vi "Positioncontrol_twomotor_pid_MotorID.vi"() -> ()   [LabVIEW 2014]
uses:
  <vilib>/rvi/FXPMathLib/FxpSinAndCos/subVIs/nifxpmath_SinAndCos_SimConfig.ctl
  <vilib>/rvi/Emulation/niFpgaGetClockAttributes.vi
  <vilib>/rvi/Emulation/niFpgaSctlEmulationGetInTimedLoop.vi
  <vilib>/rvi/Emulation/niFpgaEmulationReportErrorSimple.vi
  <vilib>/rvi/Emulation/niFpgaProcessEmulError.vi
  <vilib>/rvi/FXPMathLib/FxpSinAndCos/simVIs/DllFxpSinAndCosTemp_sub.vi
  <vilib>/rvi/Emulation/niFpgaCriticalErrorInLSC.vi
  <vilib>/rvi/eio/common/nirviEmuTemplateMethod_errors.vi
  <vilib>/rvi/interface/RandomDataEmulation/nirviRandomDataMultiElementFPGAFIFO.vi
  <instcachedir>/0/nirviRandomDataMultiElementFPGAFIFO_AD0CFC12EF974623A9C2E4184BC062B2.lvgen/nirviRandomDataMultiElementFPGAFIFO_AD0CFC12EF974623A9C2E4184BC062B2_004.vi
  <vilib>/rvi/interface/RandomDataEmulation/niFpgaRandomDataHandleErrors.vi
  <vilib>/rvi/FXPMathLib/FxpSinAndCos/XNode/nifxpmath_SinAndCos.xnode
  <vilib>/eio/EIONode/EIONode.xnode
  <vilib>/rvi/FXPMathLib/FxpMul/XNode/nifxpmath_Multiplier.xnode
  <vilib>/rvi/FXPMathLib/FxpSub/XNode/nifxpmath_Sub.xnode
  <vilib>/rvi/FXPMathLib/FxpAdd/XNode/nifxpmath_Add.xnode
  <vilib>/rvi/Analysis/measure/butterworth/XNode/niFpgaButterworthFilter.xnode
  <vilib>/rvi/DataTransferAndStorage/Container/XNode/niFpgaContainer.xnode
  <vilib>/rvi/interface/RandomDataEmulation/nirviRandomDataFpgaMultiElementTemplate.vi
  <vilib>/rvi/FXPMathLib/sim/FxpSim.dll
panel:
  in  "Dp run":bool
  in  "Dp reset":bool
  in  "vq":fxp<+/-,20,5>
  in  "vd":fxp<+/-,20,5>
  in  "Dp stroke":fxp<+,22,7> format="%#_22g"
  in  "AI loop wait (uSec)":u8=20
  in  "x_y 2 / x_y":bool
  in  "test stop/run":bool
  out "AI samp time (us) 3":u8
  in  "scaled coefficients_xy":i32[](array[numeric])=[-955995012, 2025731616, 1001305, -1023351008, 2092954700, 1034533]
  in  "scaled coefficients_xyd":i32[](array[numeric])=[-1013179863, 2085891919, 257442, -1048234864, 2120929620, 261767]
  in  "filter reset 2":bool
  out "AI diff samp time (us) 2":u8
  in  "AI diff loop wait (uSec) 2":u32
  out "Dy_d 2":fxp<+/-,25,15>
  out "Dp_d 2":fxp<+/-,25,15>
  in  "scaled coefficients_Dpd":i32[](array[numeric])=[780119100, 146811362]
  in  "scaled coefficients_Dyd":i32[](array[numeric])=[780119100, 146811362]
  in  "scaled coefficients_xpd":i32[](array[numeric])=[780119100, 146811362]
  out "xp_d 2":fxp<+/-,25,15>
  out "xy_d 2":fxp<+/-,25,15>
  out "AI samp time (us) 2":u8
  out "x_p 2":fxp<+/-,30,6> format="%.40g"
  in  "Linear Sensor Reset_y 2":bool
  out "x_y 2":fxp<+/-,30,6>
  in  "scaled coefficients_xp":i32[](array[numeric])=[1008310688, 32715568]
  in  "fyr_sin/cons":bool
  in  "fpr_sin/cons":bool
  in  "Sin_magnitude":fxp<+/-,12,8>
  in  "Sin_offset":fxp<+/-,12,8>
  out "fyr_sin":fxp<+/-,22,7> format="%.18g"
  out "fpr_sin":fxp<+/-,22,7> format="%.18g"
  in  "Sin_period(sec)":fxp<+,10,8> format="%.21g"
  in  "Time_reset":bool
  in  "coe_ini":bool
  out "fpt_i":fxp<+/-,25,11>
  out "fyt_i":fxp<+/-,25,11>
  out "time now":fxp<+/-,41,11>
  in  "D_comp/tune_p":bool
  in  "D_comp/tune_y":bool
  in  "kp t":fxp<+,15,8>
  in  "kp c":fxp<+,15,8>
  in  "Kpp gain":fxp<+,27,10>=0.40625
  in  "Kpp slope gain":fxp<+,20,1>=0.40625
  in  "Kdp 2":fxp<+,27,10>
  in  "Kip 2":fxp<+,27,10>
  in  "I_comp/tune_p":bool
  out "Kpp":fxp<+,12,6>
  out "Kdp":fxp<+,34,10> format="%.25g"
  out "Kip":fxp<+,27,10> format="%.21g"
  in  "tolerance_fp":fxp<+,12,2>=1.0
  in  "viscous_cons_p":fxp<+/-,20,10>
  in  "fcp":fxp<+/-,15,6>
  in  "fvp":fxp<+,20,12>
  in  "fv_coeff. p":fxp<+,13,1>
  in  "Dp_d_tol":fxp<+,20,12>
  in  "fstp":fxp<+/-,15,6>
  out "fpr":fxp<+/-,22,7> format="%.18g"
  out "Friction comp_p":fxp<+/-,20,10>
  out "Fp_PID":fxp<+/-,20,10>
  out "fp_tilde":fxp<+/-,26,11>
  out "xp_d":fxp<+/-,25,15>
  out "fpt_d":fxp<+/-,25,15>
  out "Dp_d":fxp<+/-,25,15>
  out "vd_p_F":fxp<+/-,20,5>
  out "vq_p_F":fxp<+/-,20,5> format="%.57g"
  in  "Stop motor_p":bool
  out "va_p":fxp<+/-,20,5> format="%.21g"
  out "vb_p":fxp<+/-,20,5> format="%.21g"
  out "omega_p":fxp<+/-,20,9>
  in  "Encoder Reset_p":bool
  out "Encoder Position_p":i32
  out "rad(NrTheta)_p":fxp<+/-,33,18> format="%.21g"
  out "Dp(mm)":fxp<+/-,22,7>
  in  "viscous_cons_y":fxp<+/-,20,10>
  in  "I_comp/tune_y":bool
  in  "fsty":fxp<+/-,15,6>
  out "Dy_d":fxp<+/-,25,15>
  out "fyr":fxp<+/-,22,7> format="%.18g"
  in  "Dy_d_tol":fxp<+,20,12>
  out "fy_tilde":fxp<+/-,26,11>
  out "fyt_d":fxp<+/-,25,15>
  in  "Kiy 2":fxp<+,27,10>
  in  "Kdy 2":fxp<+,27,10>
  in  "ky c":fxp<+,15,8>
  in  "ky t":fxp<+,15,8>
  out "Kiy":fxp<+,27,10> format="%.21g"
  in  "Kpy slope gain":fxp<+,20,1>=0.40625
  in  "Kpy gain":fxp<+,27,10>=0.40625
  in  "fv_coeff. y":fxp<+,13,1>
  out "Friction comp_y":fxp<+/-,20,10>
  in  "fcy":fxp<+/-,15,6>
  in  "fvy":fxp<+,20,12>
  out "xy_d":fxp<+/-,25,15>
  out "AI samp time (us)":u8
  out "x_p":fxp<+/-,30,6> format="%.40g"
  in  "Linear Sensor Reset_y":bool
  in  "kp":fxp<+,15,8>
  out "fp":fxp<+/-,20,10>
  in  "ky":fxp<+,15,8>
  out "fy":fxp<+/-,20,10>
  out "x_y":fxp<+/-,30,6> format="%.15g"
  out "Kdy":fxp<+,34,10> format="%.25g"
  out "Kpy":fxp<+,12,6>
  out "Fy_PID":fxp<+/-,20,10>
  in  "tolerance_fy":fxp<+,12,2>=1.0
  in  "Encoder Reset_y":bool
  out "Encoder Position_y":i32
  out "rad(NrTheta)_y":fxp<+/-,33,18> format="%.21g"
  out "Dy(mm)":fxp<+/-,22,7>
  out "omega_y":fxp<+/-,20,9>
  out "vq_y_F":fxp<+/-,20,5> format="%.57g"
  out "vd_y_F":fxp<+/-,20,5>
  in  "Stop motor_y":bool
  out "va_y":fxp<+/-,20,5> format="%.21g"
  out "vb_y":fxp<+/-,20,5> format="%.21g"
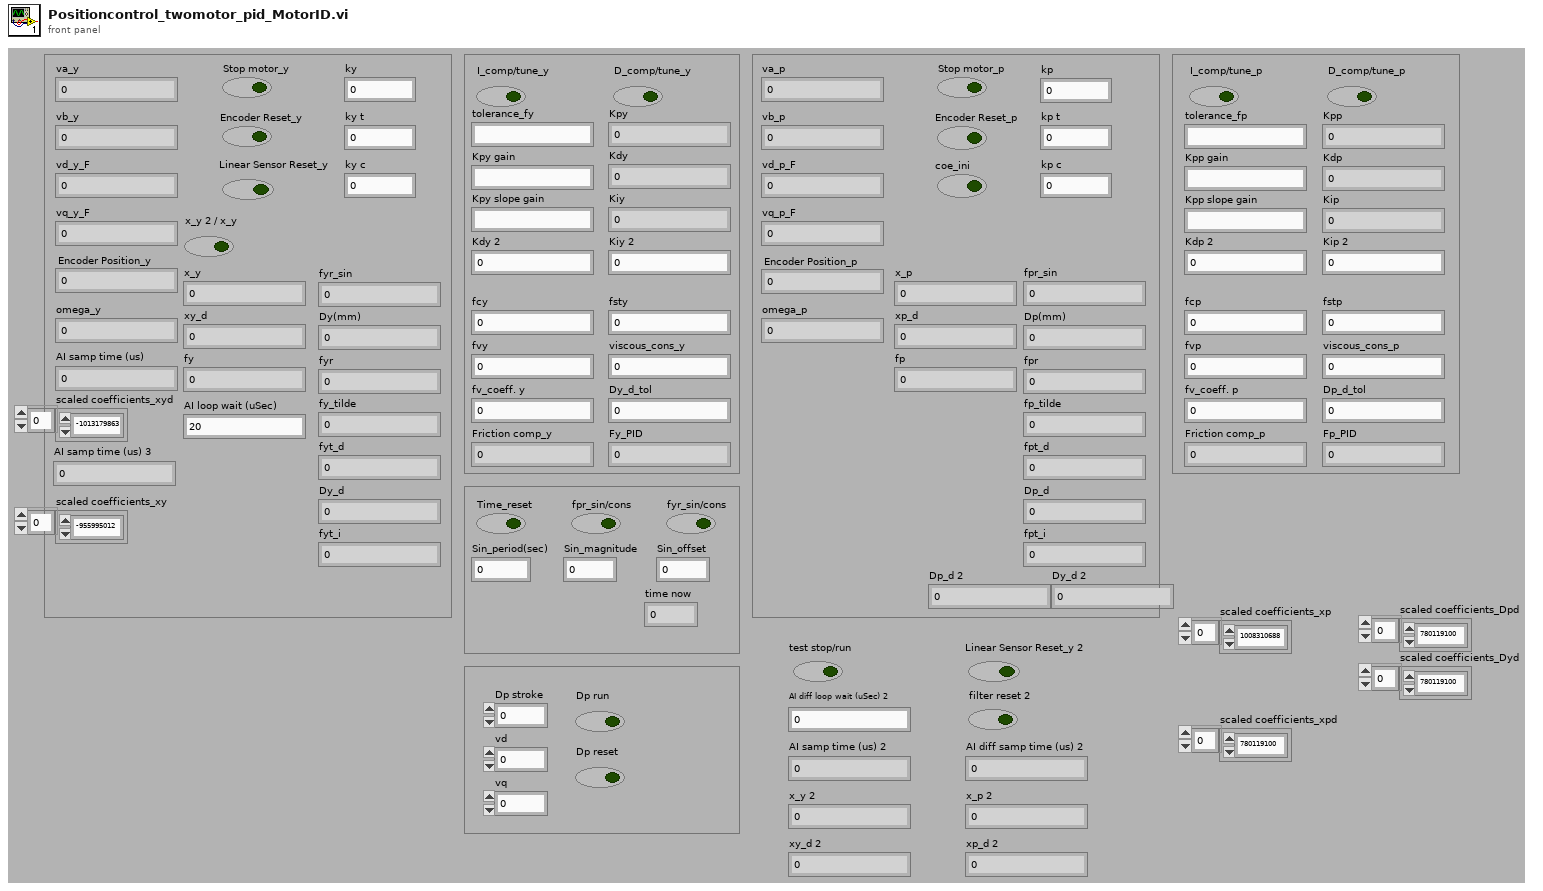
[diagram p1: front panel]
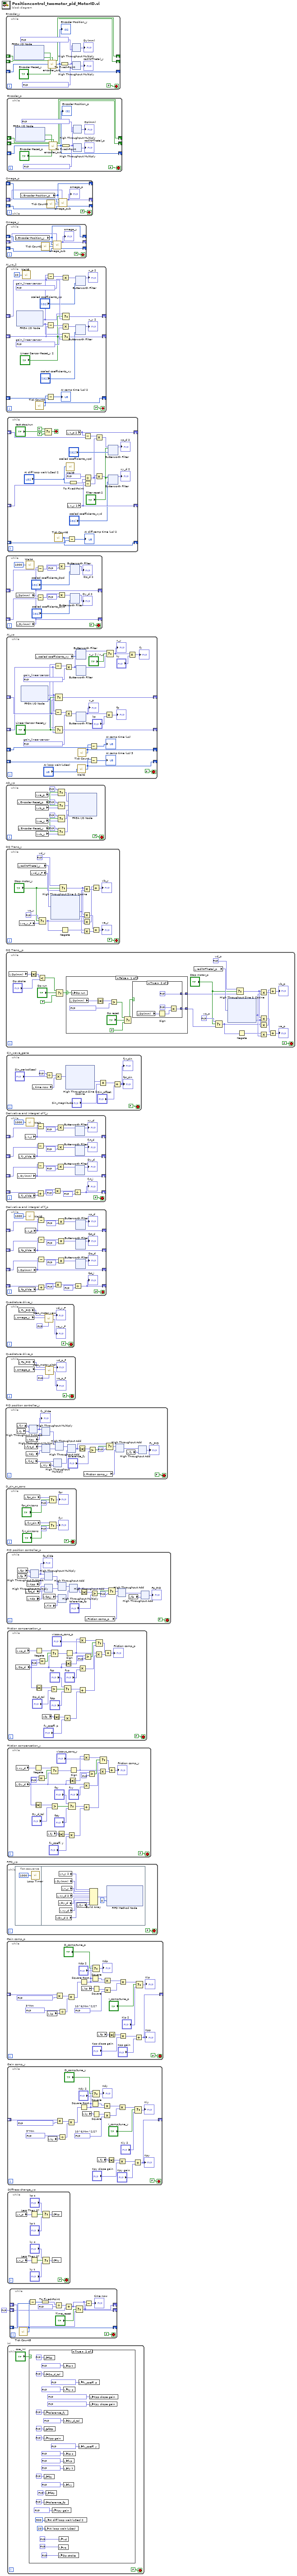
[diagram p0: block diagram]
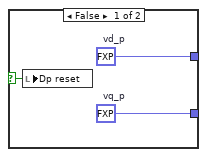
[diagram p3: hidden frame]
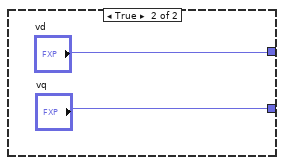
[diagram p4: hidden frame]
diagram:
  n1 = while "PID position controller_y" {
    stop <- FALSE stop-if-true
    n2 = local read "fyr"() -> (w15:fxp<+/-,22,7>)
    n3 = local read "fy"() -> (w2:fxp<+/-,20,10>)
    n4 = local read "fyt_d"() -> (w11:fxp<+/-,25,15>)
    n5 = local read "fyt_i"() -> (w9:fxp<+/-,25,11>)
    n6 = local read "Kpy"() -> (w13:fxp<+,12,6>)
    n7 = local read "Kdy"() -> (w12:fxp<+,34,10>)
    n8 = xnode "High Throughput Subtract"("x"=w15, "y"=w2) -> ("x-y"=w14:fxp<+/-,26,11>)
    "fy_tilde" <- w14
    n9 = local read "Kiy"() -> (w10:fxp<+,27,10>)
    n10 = xnode ("High Throughput Multiply")("x"=w14, "y"=w13) -> ("x*y"=w8:fxp<+/-,38,17>)
    n11 = xnode ("High Throughput Multiply")("x"=w11, "y"=w12) -> ("x*y"=w7:fxp<+/-,59,25>)
    n12 = xnode ("High Throughput Multiply")("x"=w9, "y"=w10) -> ("x*y"=w6:fxp<+/-,52,21>)
    n13 = xnode ("High Throughput Add")("x"=w8, "y"=w7) -> ("x+y"=w5:fxp<+/-,60,26>)
    n14 = xnode ("High Throughput Add")("x"=w5, "y"=w6) -> ("x+y"=w4:fxp<+/-,20,10>)
    n15 = Absolute Value(x=w4) -> (abs(x)=w22:fxp<+,20,10>)
    n16 = local read "Friction comp_y"() -> (w16:fxp<+/-,20,10>)
    n17 = Greater?(x=w22, y="tolerance_fy") -> (0:w21:bool)
    n18 = Select(t=w4, s=w21, f=fxp<+/-,20,10> 0.0) -> (s? t:f=w18:fxp<+/-,20,10>)
    n19 = xnode ("High Throughput Add")("x"=w18, "y"=w16) -> ("x+y"=w17:fxp<+/-,20,10>)
    n20 = local read "fy"() -> (w19:fxp<+/-,20,10>)
    n21 = xnode ("High Throughput Add")("x"=w17, "y"=w19) -> ("x+y"=→"Fy_PID":fxp<+/-,20,10>)
  }
  n22 = while "Encoder_y" {
    shift-right: [w38] -> _
    shift-left: _ -> [w36]
    shift-right: [w37] -> _
    shift-left: _ -> [w35]
    shift-right: [w25] -> _
    shift-left: _ -> [w31]
    stop <- FALSE stop-if-true
    n23 = xnode "FPGA I/O Node"() -> ("Mod3/DIO2"=w34:bool, "Mod3/DIO3"=w33:bool)  [unwired: 2 in, 2 out]
    n24 = call "encoder_sub.vi"("A_pre"=w36, "B_pre"=w35, "Encoder Position_pre"=w31, "A input"=w34, "Encoder Position Reset"="Encoder Reset_y", "B input"=w33) -> ("A"=w38:bool, "B"=w37:bool, "Encoder Position (Counts)"=w25:i32)  [unwired: 19 in]
    "Encoder Position_y" <- w25
    n25 = To Fixed-Point(number=w25) -> (fixed-point=w28:fxp<+/-,18,18>)  [unwired: 1 in]
    n26 = xnode ("High Throughput Multiply")("x"=w28, "y"=fxp<+/-,15,-9> -0.0006049871444702148) -> ("x*y"=→"Dy(mm)":fxp<+/-,21,6>)
    n27 = xnode ("High Throughput Multiply")("x"=w28, "y"=fxp<+,24,0> 0.02499997615814209) -> ("x*y"=→"rad(NrTheta)_y":fxp<+/-,33,18>)
  }
  n28 = while "Omega_p" {
    shift-right: [w47] -> _
    shift-left: _ -> [w46]
    shift-right: [w45] -> _
    shift-left: _ -> [w44]
    shift-right: [w42] -> _
    shift-left: _ -> [w43]
    stop <- FALSE stop-if-true
    n29 = local read "Encoder Position_p"() -> (w47:i32)
    n30 = call "Tick Count3"() -> ("Tick Count(Ticks)"=w40:u32)
    n31 = call "omega_sub.vi"("omega_pre"=w43, "ticks_m_pre"=w44, "ticks"=w40, "count_pre"=w46, "count"=w47) -> ("ticks_m"=w45:u32, "omega"=w42:fxp<+/-,20,9>)  [unwired: 5 in]
    "omega_p" <- w42
  }
  n32 = while "Omega_y" {
    shift-right: [w55] -> _
    shift-left: _ -> [w54]
    shift-right: [w53] -> _
    shift-left: _ -> [w52]
    shift-right: [w50] -> _
    shift-left: _ -> [w51]
    stop <- FALSE stop-if-true
    n33 = local read "Encoder Position_y"() -> (w55:i32)
    n34 = call "Tick Count2"() -> ("Tick Count(Ticks)"=w48:u32)
    n35 = call "omega_sub.vi"("omega_pre"=w51, "ticks_m_pre"=w52, "ticks"=w48, "count_pre"=w54, "count"=w55) -> ("ticks_m"=w53:u32, "omega"=w50:fxp<+/-,20,9>)  [unwired: 5 in]
    "omega_y" <- w50
  }
  n36 = while "AI_yp_2" {
    shift-right: [w76] -> _
    shift-left: _ -> [w77]
    shift-right: [w73] -> _
    shift-left: _ -> [w74]
    shift-right: [w71] -> _
    shift-left: _ -> [w70]
    stop <- FALSE stop-if-true
    w62 = fxp<+,25,5> 1.4694995880126953  # gain_linear sensor
    w67 = fxp<+,25,5> 1.5044002532958984  # gain_linear sensor
    n37 = xnode "FPGA I/O Node"() -> ("Mod1/AI0"=w72:fxp<+/-,20,5>, "Mod1/AI1"=w69:fxp<+/-,20,5>)  [unwired: 3 in, 3 out]
    n38 = call "Wait8"("Count(uSec)"=u8 20) -> ()  [unwired: 1 out]
    n39 = call "Tick Count4"() -> ("Tick Count(uSec)"=w76:u8)
    n40 = Subtract(x=w72, y=w74) -> (x-y=w66:fxp<+/-,21,6>)
    n41 = Subtract(x=w69, y=w70) -> (x-y=w68:fxp<+/-,21,6>)
    n42 = Subtract(x=w76, y=w77) -> (x-y=→"AI samp time (us) 2":u8)
    n43 = Multiply(x=w66, y=w62) -> (x*y=w64:fxp<+/-,30,6>)
    n44 = Multiply(x=w68, y=w67) -> (x*y=w63:fxp<+/-,30,6>)
    n45 = Select(t=w72, s="Linear Sensor Reset_y 2", f=w74) -> (s? t:f=w73:fxp<+/-,20,5>)
    n46 = Select(t=w69, s="Linear Sensor Reset_y 2", f=w70) -> (s? t:f=w71:fxp<+/-,20,5>)
    n47 = xnode "Butterworth Filter"("input data"=w64, "scaled coefficients"="scaled coefficients_xp") -> ("output data"=→"x_p 2":fxp<+/-,30,6>)  [unwired: 1 in]
    n48 = xnode "Butterworth Filter"("input data"=w63, "scaled coefficients"="scaled coefficients_xy") -> ("output data"=→"x_y 2":fxp<+/-,30,6>)  [unwired: 1 in]
  }
  n49 = while {
    shift-right: [w100] -> _
    shift-left: _ -> [w101]
    shift-right: [w98] -> _
    shift-left: _ -> [w99]
    stop <- FALSE stop-if-true
    n50 = local read "Dp(mm)"() -> (w100:fxp<+/-,22,7>)
    n51 = local read "Dy(mm)"() -> (w98:fxp<+/-,22,7>)
    n52 = call "Wait4"("Count(uSec)"=u32 1000 ("Count(mSec)")) -> ()  [unwired: 1 out]
    n53 = Subtract(x=w100, y=w101) -> (x-y=w106:fxp<+/-,23,8>)
    n54 = Subtract(x=w98, y=w99) -> (x-y=w103:fxp<+/-,23,8>)
    n55 = Multiply(x=w106, y=fxp<+,10,10> 1000.0) -> (x*y=w107:fxp<+/-,25,15>)
    n56 = Multiply(x=w103, y=fxp<+,10,10> 1000.0) -> (x*y=w102:fxp<+/-,25,15>)
    n57 = xnode "Butterworth Filter"("input data"=w107, "scaled coefficients"="scaled coefficients_Dpd") -> ("output data"=→"Dp_d 2":fxp<+/-,25,15>)  [unwired: 1 in]
    n58 = xnode "Butterworth Filter"("input data"=w102, "scaled coefficients"="scaled coefficients_Dyd") -> ("output data"=→"Dy_d 2":fxp<+/-,25,15>)  [unwired: 1 in]
  }
  n59 = while "AO_yp" {
    stop <- FALSE stop-if-true
    n60 = local read "Encoder Reset_p"() -> (w139:bool)
    n61 = local read "Encoder Reset_y"() -> (w128:bool)
    n62 = local read "va_p"() -> (w138:fxp<+/-,20,5>)
    n63 = local read "vb_p"() -> (w137:fxp<+/-,20,5>)
    n64 = local read "va_y"() -> (w129:fxp<+/-,20,5>)
    n65 = local read "vb_y"() -> (w130:fxp<+/-,20,5>)
    n66 = Select(t=fxp<+/-,20,5> 5.0 ("Mod2/AO4"), s=w139, f=w138) -> (s? t:f=w134:fxp<+/-,20,5>)
    n67 = Select(t=fxp<+/-,20,5> 0.0 ("Mod2/AO4"), s=w139, f=w137) -> (s? t:f=w133:fxp<+/-,20,5>)
    n68 = Select(t=fxp<+/-,20,5> 5.0 ("Mod2/AO4"), s=w128, f=w129) -> (s? t:f=w127:fxp<+/-,20,5>)
    n69 = Select(t=fxp<+/-,20,5> 0.0 ("Mod2/AO4"), s=w128, f=w130) -> (s? t:f=w126:fxp<+/-,20,5>)
    n70 = xnode "FPGA I/O Node"("Mod2/AO0"=w134, "Mod2/AO1"=w133, "Mod2/AO2"=w127, "Mod2/AO3"=w126) -> ()  [unwired: 4 in, 4 out]
  }
  n71 = while "DQ Trans_y" {
    stop <- FALSE stop-if-true
    w146 = fxp<+/-,20,5> 0.0  # vq_y
    w144 = fxp<+/-,20,5> 0.0  # vd_y
    n72 = local read "rad(NrTheta)_y"() -> (w157:fxp<+/-,33,18>)
    n73 = local read "vq_y_F"() -> (w142:fxp<+/-,20,5>)
    n74 = local read "vd_y_F"() -> (w143:fxp<+/-,20,5>)
    n75 = Select(t=w146, s="Stop motor_y", f=w142) -> (s? t:f=w147:fxp<+/-,20,5>)
    n76 = xnode "High Throughput Sine & Cosine"("x (pi)"=w157) -> ("sin(x)"=w148:fxp<+/-,17,2>, "cos(x)"=w149:fxp<+/-,17,2>)
    n77 = Select(t=w144, s="Stop motor_y", f=w143) -> (s? t:f=w145:fxp<+/-,20,5>)
    n78 = Negate(x=w147) -> (-x=w156:fxp<+/-,21,6>)
    n79 = Multiply(x=w145, y=w148) -> (x*y=w152:fxp<+/-,20,5>)
    n80 = Multiply(x=w145, y=w149) -> (x*y=w155:fxp<+/-,20,5>)
    n81 = Multiply(x=w147, y=w149) -> (x*y=w151:fxp<+/-,20,5>)
    n82 = Multiply(x=w156, y=w148) -> (x*y=w154:fxp<+/-,20,5>)
    n83 = Add(x=w151, y=w152) -> (x+y=→"vb_y":fxp<+/-,20,5>)
    n84 = Add(x=w155, y=w154) -> (x+y=→"va_y":fxp<+/-,20,5>)
  }
  n85 = while "DQ Trans__p" {
    stop <- FALSE stop-if-true
    w203 = fxp<+/-,20,5> 0.0  # vq_p
    w201 = fxp<+/-,20,5> 0.0  # vd_p
    n86 = local read "Dp(mm)"() -> (w190:fxp<+/-,22,7>)
    n87 = Absolute Value(x=w190) -> (abs(x)=w189:fxp<+,22,7>)
    n88 = Less?(x=w189, y="Dp stroke") -> (x < y?=w193:bool)
    n89 = Select(t=w193, s="Dp run", f=FALSE) -> (s? t:f=w192:bool)
    n90 = case shown="False" w192 {
      selector: w192 -> [w223 _]
      tunnel: [w214 "vd"] -> w196
      tunnel: [w215 "vq"] -> w195
      frame False {
        n91 = local read "Dp(mm)"() -> (w222:fxp<+/-,22,7>)
        n92 = local write "Dp run"(w223) -> ()
        n93 = Absolute Value(x=w222) -> (abs(x)=w221:fxp<+,22,7>)
        n94 = Greater?(x=w221, y=fxp<+,22,7> 0.010009765625) -> (0:w218:bool)
        n95 = Select(t=w218, s="Dp reset", f=FALSE) -> (s? t:f=w217:bool)
        n96 = case shown="True" w217 {
          selector: w217 -> [w224 _]
          tunnel: [w226 w228] -> w215
          tunnel: [w225 fxp<+/-,20,5> 5.0] -> w214
          frame False {
            w226 = fxp<+/-,20,5> 0.0  # vq_p
            w225 = fxp<+/-,20,5> 0.0  # vd_p
            n97 = local write "Dp reset"(w224) -> ()
          }
          frame True {
            n98 = local read "Dp(mm)"() -> (w231:fxp<+/-,22,7>)
            n99 = Sign(1:w231) -> (0:w229:fxp<+/-,2,2>)
            n100 = Multiply(x=fxp<+/-,19,4> 5.0, y=w229) -> (x*y=w228:fxp<+/-,20,5>)
          }
        }
      }
      frame True {
      }
    }
    n101 = local read "rad(NrTheta)_p"() -> (w212:fxp<+/-,33,18>)
    n102 = Select(t=w203, s="Stop motor_p", f=w195) -> (s? t:f=w204:fxp<+/-,20,5>)
    n103 = xnode "High Throughput Sine & Cosine"("x (pi)"=w212) -> ("sin(x)"=w205:fxp<+/-,17,2>, "cos(x)"=w206:fxp<+/-,17,2>)
    n104 = Select(t=w201, s="Stop motor_p", f=w196) -> (s? t:f=w202:fxp<+/-,20,5>)
    n105 = Negate(x=w204) -> (-x=w211:fxp<+/-,21,6>)
    n106 = Multiply(x=w202, y=w205) -> (x*y=w208:fxp<+/-,20,5>)
    n107 = Multiply(x=w202, y=w206) -> (x*y=w210:fxp<+/-,20,5>)
    n108 = Multiply(x=w204, y=w206) -> (x*y=w207:fxp<+/-,20,5>)
    n109 = Multiply(x=w211, y=w205) -> (x*y=w209:fxp<+/-,20,5>)
    n110 = Add(x=w207, y=w208) -> (x+y=→"vb_p":fxp<+/-,20,5>)
    n111 = Add(x=w210, y=w209) -> (x+y=→"va_p":fxp<+/-,20,5>)
  }
  n112 = while "Derivative and intergral of f_y" {
    shift-right: [w285] -> _
    shift-left: _ -> [w284]
    shift-right: [w281] -> _
    shift-left: _ -> [w282]
    shift-right: [w274] -> _
    shift-left: _ -> [w273]
    shift-right: [w266] -> _
    shift-left: _ -> [w267]
    stop <- FALSE stop-if-true
    n113 = local read "Dy(mm)"() -> (w274:fxp<+/-,22,7>)
    n114 = local read "fy_tilde"() -> (w281:fxp<+/-,26,11>)
    n115 = local read "fy_tilde"() -> (w268:fxp<+/-,26,11>)
    n116 = local read "x_y"() -> (w285:fxp<+/-,30,6>)
    n117 = call "Wait"("Count(uSec)"=u32 1000 ("Count(mSec)")) -> ()  [unwired: 1 out]
    n118 = Subtract(x=w285, y=w284) -> (x-y=w287:fxp<+/-,31,7>)
    n119 = Subtract(x=w281, y=w282) -> (x-y=w278:fxp<+/-,27,12>)
    n120 = Subtract(x=w274, y=w273) -> (x-y=w276:fxp<+/-,23,8>)
    n121 = Add(x=w267, y=w268) -> (x+y=w269:fxp<+/-,27,12>)
    n122 = Multiply(x=w269, y=fxp<+/-,22,12> 0.5) -> (x*y=w271:fxp<+/-,25,15>)
    n123 = Multiply(x=w287, y=fxp<+,10,10> 1000.0) -> (x*y=w286:fxp<+/-,25,15>)
    n124 = Multiply(x=w278, y=fxp<+,10,10> 1000.0) -> (x*y=w280:fxp<+/-,25,15>)
    n125 = Multiply(x=w276, y=fxp<+,10,10> 1000.0) -> (x*y=w265:fxp<+/-,25,15>)
    n126 = Divide(x=w271, y=fxp<+/-,25,15> 1000.0) -> (x/y=w266:fxp<+/-,25,11>)
    "fyt_i" <- w266
    n127 = xnode "Butterworth Filter"("input data"=w286) -> ("output data"=→"xy_d":fxp<+/-,25,15>)  [unwired: 2 in]
    n128 = xnode "Butterworth Filter"("input data"=w280) -> ("output data"=→"fyt_d":fxp<+/-,25,15>)  [unwired: 2 in]
    n129 = xnode "Butterworth Filter"("input data"=w265) -> ("output data"=→"Dy_d":fxp<+/-,25,15>)  [unwired: 2 in]
  }
  n130 = while "Derivative and intergral of f_p" {
    shift-right: [w333] -> _
    shift-left: _ -> [w332]
    shift-right: [w329] -> _
    shift-left: _ -> [w330]
    shift-right: [w322] -> _
    shift-left: _ -> [w321]
    shift-right: [w314] -> _
    shift-left: _ -> [w315]
    stop <- FALSE stop-if-true
    n131 = local read "Dp(mm)"() -> (w322:fxp<+/-,22,7>)
    n132 = local read "fp_tilde"() -> (w329:fxp<+/-,26,11>)
    n133 = local read "fp_tilde"() -> (w320:fxp<+/-,26,11>)
    n134 = local read "x_p"() -> (w333:fxp<+/-,30,6>)
    n135 = call "Wait3"("Count(uSec)"=u32 1000 ("Count(mSec)")) -> ()  [unwired: 1 out]
    n136 = Subtract(x=w333, y=w332) -> (x-y=w335:fxp<+/-,31,7>)
    n137 = Subtract(x=w329, y=w330) -> (x-y=w326:fxp<+/-,27,12>)
    n138 = Subtract(x=w322, y=w321) -> (x-y=w324:fxp<+/-,23,8>)
    n139 = Add(x=w315, y=w320) -> (x+y=w319:fxp<+/-,27,12>)
    n140 = Multiply(x=w319, y=fxp<+/-,22,12> 0.5) -> (x*y=w317:fxp<+/-,25,15>)
    n141 = Multiply(x=w335, y=fxp<+,10,10> 1000.0) -> (x*y=w334:fxp<+/-,25,15>)
    n142 = Multiply(x=w326, y=fxp<+,10,10> 1000.0) -> (x*y=w328:fxp<+/-,25,15>)
    n143 = Multiply(x=w324, y=fxp<+,10,10> 1000.0) -> (x*y=w313:fxp<+/-,25,15>)
    n144 = Divide(x=w317, y=fxp<+/-,25,15> 1000.0) -> (x/y=w314:fxp<+/-,25,11>)
    "fpt_i" <- w314
    n145 = xnode "Butterworth Filter"("input data"=w334) -> ("output data"=→"xp_d":fxp<+/-,25,15>)  [unwired: 2 in]
    n146 = xnode "Butterworth Filter"("input data"=w328) -> ("output data"=→"fpt_d":fxp<+/-,25,15>)  [unwired: 2 in]
    n147 = xnode "Butterworth Filter"("input data"=w313) -> ("output data"=→"Dp_d":fxp<+/-,25,15>)  [unwired: 2 in]
  }
  n148 = while "Quadrature drive_y" {
    stop <- FALSE stop-if-true
    n149 = local read "omega_y"() -> (w363:fxp<+/-,20,9>)
    n150 = local read "Fy_PID"() -> (w364:fxp<+/-,20,10>)
    n151 = call "step_motor_yaw.vi"("F_Threshold"=fxp<+,12,12> 10.0, "omega_y"=w363, "F"=w364) -> ("vq_F"=→"vq_y_F":fxp<+/-,20,5>, "vd_F"=→"vd_y_F":fxp<+/-,20,5>)  [unwired: 7 in]
  }
  n152 = while "Quadrature drive_p" {
    stop <- FALSE stop-if-true
    n153 = local read "omega_p"() -> (w368:fxp<+/-,20,9>)
    n154 = local read "Fp_PID"() -> (w370:fxp<+/-,20,10>)
    n155 = call "step_motor_pitch.vi"("F_Threshold"=fxp<+,12,12> 10.0, "omega_p"=w368, "F"=w370) -> ("vq_F"=→"vq_p_F":fxp<+/-,20,5>, "vd_F"=→"vd_p_F":fxp<+/-,20,5>)  [unwired: 7 in]
  }
  n156 = while "D_sin_or_cons" {
    stop <- FALSE stop-if-true
    n157 = local read "fpr_sin"() -> (w376:fxp<+/-,22,7>)
    n158 = local read "fyr_sin"() -> (w375:fxp<+/-,22,7>)
    n159 = Select(t=w376, s="fpr_sin/cons", f=fxp<+/-,22,7> 0.0) -> (s? t:f=→"fpr":fxp<+/-,22,7>)
    n160 = Select(t=w375, s="fyr_sin/cons", f=fxp<+/-,22,7> 0.0) -> (s? t:f=→"fyr":fxp<+/-,22,7>)
  }
  n161 = while "AI_yp" {
    shift-right: [w410] -> _
    shift-left: _ -> [w411]
    shift-right: [w406] -> _
    shift-left: _ -> [w407]
    shift-right: [w401] -> _
    shift-left: _ -> [w400]
    shift-right: [w389] -> _
    shift-left: _ -> [w388]
    stop <- FALSE stop-if-true
    w390 = fxp<+,25,5> 1.4694995880126953  # gain_linear sensor
    w397 = fxp<+,25,5> 1.5044002532958984  # gain_linear sensor
    n162 = xnode "FPGA I/O Node"() -> ("Mod1/AI0"=w403:fxp<+/-,20,5>, "Mod1/AI1"=w399:fxp<+/-,20,5>)  [unwired: 3 in, 3 out]
    n163 = local read "scaled coefficients_xy"() -> (w382:i32[])
    n164 = Subtract(x=w399, y=w400) -> (x-y=w398:fxp<+/-,21,6>)
    n165 = Subtract(x=w403, y=w407) -> (x-y=w394:fxp<+/-,21,6>)
    n166 = Select(t=w403, s="Linear Sensor Reset_y", f=w407) -> (s? t:f=w406:fxp<+/-,20,5>)
    n167 = Select(t=w399, s="Linear Sensor Reset_y", f=w400) -> (s? t:f=w401:fxp<+/-,20,5>)
    n168 = Multiply(x=w394, y=w390) -> (x*y=w392:fxp<+/-,30,6>)
    n169 = Multiply(x=w398, y=w397) -> (x*y=w381:fxp<+/-,30,6>)
    n170 = xnode "Butterworth Filter"("input data"=w381, "scaled coefficients"=w382) -> ("output data"=w384:fxp<+/-,30,6>)  [unwired: 1 in]
    n171 = xnode "Butterworth Filter"("input data"=w381) -> ("output data"=w383:fxp<+/-,30,6>)  [unwired: 2 in]
    n172 = xnode "Butterworth Filter"("input data"=w392) -> ("output data"=w391:fxp<+/-,30,6>)  [unwired: 2 in]
    "x_p" <- w391
    n173 = call "Wait2"("Count(uSec)"="AI loop wait (uSec)") -> ("Tick Count(uSec)"=w389:u8)
    n174 = call "Tick Count"() -> ("Tick Count(uSec)"=w410:u8)
    n175 = Subtract(x=w410, y=w411) -> (x-y=→"AI samp time (us)":u8)
    n176 = Subtract(x=w389, y=w388) -> (x-y=→"AI samp time (us) 3":u8)
    n177 = Multiply(x=w391, y="kp") -> (x*y=→"fp":fxp<+/-,20,10>)
    n178 = Select(t=w384, s="x_y 2 / x_y", f=w383) -> (s? t:f=w385:fxp<+/-,30,6>)
    "x_y" <- w385
    n179 = Multiply(x=w385, y="ky") -> (x*y=→"fy":fxp<+/-,20,10>)
  }
  n180 = while "Sin_wave_gene" {
    stop <- FALSE stop-if-true
    n181 = local read "time now"() -> (w445:fxp<+/-,41,11>)
    n182 = Divide(x=fxp<+,10,8> 2.0, y="Sin_period(sec)") -> (x/y=w444:fxp<+/-,20,11>)
    n183 = Multiply(x=w444, y=w445) -> (x*y=w443:fxp<+/-,25,11>)
    n184 = xnode "High Throughput Sine & Cosine"("x (pi)"=w443) -> ("sin(x)"=w441:fxp<+/-,17,2>)  [unwired: 1 out]
    n185 = Multiply(x=w441, y="Sin_magnitude") -> (x*y=w439:fxp<+/-,20,8>)
    n186 = Add(x=w439, y="Sin_offset") -> (x+y=→"fyr_sin" →"fpr_sin":fxp<+/-,22,7>)
  }
  n187 = while "PID position controller_p" {
    stop <- FALSE stop-if-true
    n188 = local read "fpr"() -> (w488:fxp<+/-,22,7>)
    n189 = local read "fp"() -> (w477:fxp<+/-,20,10>)
    n190 = local read "fpt_d"() -> (w491:fxp<+/-,25,15>)
    n191 = local read "Kpp"() -> (w489:fxp<+,12,6>)
    n192 = local read "Kdp"() -> (w490:fxp<+,34,10>)
    n193 = xnode "High Throughput Subtract"("x"=w488, "y"=w477) -> ("x-y"=w484:fxp<+/-,26,11>)
    "fp_tilde" <- w484
    n194 = local read "fpt_i"() -> (w493:fxp<+/-,25,11>)
    n195 = xnode ("High Throughput Multiply")("x"=w484, "y"=w489) -> ("x*y"=w494:fxp<+/-,38,17>)
    n196 = xnode ("High Throughput Multiply")("x"=w491, "y"=w490) -> ("x*y"=w495:fxp<+/-,59,25>)
    n197 = local read "Kip"() -> (w492:fxp<+,27,10>)
    n198 = xnode ("High Throughput Add")("x"=w494, "y"=w495) -> ("x+y"=w497:fxp<+/-,60,26>)
    n199 = xnode ("High Throughput Multiply")("x"=w493, "y"=w492) -> ("x*y"=w496:fxp<+/-,52,21>)
    n200 = xnode ("High Throughput Add")("x"=w497, "y"=w496) -> ("x+y"=w498:fxp<+/-,20,10>)
    n201 = Absolute Value(x=w498) -> (abs(x)=w485:fxp<+,20,10>)
    n202 = local read "Friction comp_p"() -> (w481:fxp<+/-,20,10>)
    n203 = Greater?(x=w485, y="tolerance_fp") -> (0:w486:bool)
    n204 = Select(t=w498, s=w486, f=fxp<+/-,20,10> 0.0) -> (s? t:f=w482:fxp<+/-,20,10>)
    n205 = xnode ("High Throughput Add")("x"=w482, "y"=w481) -> ("x+y"=w479:fxp<+/-,20,10>)
    n206 = local read "fp"() -> (w480:fxp<+/-,20,10>)
    n207 = xnode ("High Throughput Add")("x"=w479, "y"=w480) -> ("x+y"=→"Fp_PID":fxp<+/-,20,10>)
  }
  n208 = while "FIFO_yp" {
    stop <- FALSE stop-if-true
    n209 = flat-sequence {
      frame #0 {
        n210 = call "Loop Timer"("Count(uSec)"=u32 1000 ("Loop Period (usec)")) -> ()  [unwired: 1 out]
      }
      frame #1 {
        n211 = local read "Dy(mm)"() -> (w508:fxp<+/-,22,7>)
        n212 = local read "Dy_d 2"() -> (w503:fxp<+/-,25,15>)
        n213 = local read "xy_d 2"() -> (w506:fxp<+/-,25,15>)
        n214 = local read "Dy_d"() -> (w505:fxp<+/-,25,15>)
        n215 = local read "x_y 2"() -> (w511:fxp<+/-,30,6>)
        n216 = local read "xy_d"() -> (w504:fxp<+/-,25,15>)
        n217 = local read "x_y"() -> (w507:fxp<+/-,30,6>)
        n218 = local read "fyr"() -> (w502:fxp<+/-,22,7>)
        n219 = Build Array(w511, w508, w507, w506, w505, w504, w503, w502) -> (w510:fxp<+/-,39,15>[])
        n220 = xnode ("FIFO Method Node")("Element"=w510, "Timeout"=0) -> ()  [unwired: 1 in, 2 out]
      }
    }
  }
  n221 = while "Gain comp_p" {
    shift-right: [w516] -> _
    shift-left: _ -> [w535]
    stop <- FALSE stop-if-true
    w523 = fxp<+,14,7> 111.8125  # 10^6/Mm^2/27
    w538 = fxp<+,14,7> 54.6015625  # 3*Mm
    n222 = local read "kp"() -> (w537:fxp<+,15,8>)
    n223 = Multiply(x=w535, y=fxp<+,12,-6> 0.00099945068359375) -> (x*y=w534:fxp<+,24,0>)
    n224 = Divide(x=w538, y=w537) -> (x/y=w533:fxp<+,23,7>)
    n225 = Multiply(x=w534, y=w533) -> (x*y=w532:fxp<+,32,0>)
    n226 = Square Root(x=w532) -> (sqrt(x)=w519:fxp<+,26,2>)
    n227 = local read "kp"() -> (w524:fxp<+,15,8>)
    n228 = Square(x=w519) -> (x^2=w526:fxp<+,27,3>)
    n229 = Select(t=w519, s="D_comp/tune_p", f="Kdp 2") -> (s? t:f=→"Kdp":fxp<+,34,10>)
    n230 = Square(x=w524) -> (x^2=w522:fxp<+,30,16>)
    n231 = local read "fp"() -> (w529:fxp<+/-,20,10>)
    n232 = Multiply(x=w526, y=w519) -> (x*y=w525:fxp<+,27,3>)
    n233 = Multiply(x=w522, y=w523) -> (x*y=w521:fxp<+,44,20>)
    n234 = Absolute Value(x=w529) -> (abs(x)=w530:fxp<+,20,10>)
    n235 = Multiply(x=w525, y=w521) -> (x*y=w518:fxp<+,27,10>)
    n236 = Multiply(x=w530, y="Kpp slope gain") -> (x*y=w528:fxp<+,12,4>)
    n237 = Add(x=w528, y="Kpp gain") -> (x+y=w516:fxp<+,12,6>)
    "Kpp" <- w516
    n238 = Select(t=w518, s="I_comp/tune_p", f="Kip 2") -> (s? t:f=→"Kip":fxp<+,27,10>)
  }
  n239 = while "Encoder_p" {
    shift-right: [w553] -> _
    shift-left: _ -> [w551]
    shift-right: [w552] -> _
    shift-left: _ -> [w550]
    shift-right: [w540] -> _
    shift-left: _ -> [w546]
    stop <- FALSE stop-if-true
    n240 = xnode "FPGA I/O Node"() -> ("Mod3/DIO0"=w549:bool, "Mod3/DIO1"=w548:bool)  [unwired: 2 in, 2 out]
    n241 = call "encoder_sub.vi"("A_pre"=w551, "B_pre"=w550, "Encoder Position_pre"=w546, "A input"=w549, "Encoder Position Reset"="Encoder Reset_p", "B input"=w548) -> ("A"=w553:bool, "B"=w552:bool, "Encoder Position (Counts)"=w540:i32)  [unwired: 19 in]
    "Encoder Position_p" <- w540
    n242 = To Fixed-Point(number=w540) -> (fixed-point=w543:fxp<+/-,18,18>)  [unwired: 1 in]
    n243 = xnode ("High Throughput Multiply")("x"=w543, "y"=fxp<+/-,15,-9> -0.0006049871444702148) -> ("x*y"=→"Dp(mm)":fxp<+/-,21,6>)
    n244 = xnode ("High Throughput Multiply")("x"=w543, "y"=fxp<+,24,0> 0.02499997615814209) -> ("x*y"=→"rad(NrTheta)_p":fxp<+/-,33,18>)
  }
  n245 = while {
    shift-right: [w575] -> _
    shift-left: _ -> [w576]
    shift-right: [w573] -> _
    shift-left: _ -> [w574]
    shift-right: [w567] -> _
    shift-left: _ -> [w568]
    stop <- w555 stop-if-true
    n246 = Select(t=TRUE, s="test stop/run", f=FALSE) -> (s? t:f=w555:bool)
    n247 = call "Tick Count6"() -> ("Tick Count(uSec)"=w567:u8)
    n248 = call "Wait9"("Count(uSec)"="AI diff loop wait (uSec) 2") -> ()  [unwired: 1 out]
    n249 = local read "x_p 2"() -> (w575:fxp<+/-,30,6>)
    n250 = local read "x_y 2"() -> (w573:fxp<+/-,30,6>)
    n251 = Subtract(x=w567, y=w568) -> (x-y=→"AI diff samp time (us) 2":u8)
    n252 = To Fixed-Point(number="AI diff loop wait (uSec) 2") -> (fixed-point=w563:fxp<+,10,10>)  [unwired: 1 in]
    n253 = Subtract(x=w575, y=w576) -> (x-y=w578:fxp<+/-,31,7>)
    n254 = Subtract(x=w573, y=w574) -> (x-y=w577:fxp<+/-,31,7>)
    n255 = Divide(x=fxp<+,14,20> 1000000.0, y=w563) -> (x/y=w561:fxp<+,24,20>)
    n256 = Multiply(x=w578, y=w561) -> (x*y=w562:fxp<+/-,25,15>)
    n257 = Multiply(x=w577, y=w561) -> (x*y=w560:fxp<+/-,25,15>)
    n258 = xnode "Butterworth Filter"("input data"=w562, "reset"="filter reset 2", "scaled coefficients"="scaled coefficients_xpd") -> ("output data"=→"xp_d 2":fxp<+/-,25,15>)
    n259 = xnode "Butterworth Filter"("input data"=w560, "reset"="filter reset 2", "scaled coefficients"="scaled coefficients_xyd") -> ("output data"=→"xy_d 2":fxp<+/-,25,15>)
  }
  n260 = while "Friction compensation_p" {
    stop <- FALSE stop-if-true
    n261 = local read "Dp_d"() -> (w601:fxp<+/-,25,15>)
    n262 = local read "xp_d"() -> (w596:fxp<+/-,25,15>)
    n263 = Negate(x=w596) -> (-x=w595:fxp<+/-,26,16>)
    n264 = Absolute Value(x=w601) -> (abs(x)=w614:fxp<+,25,15>)
    n265 = Equal?(x=w601, y=fxp<+/-,25,15> 0.0) -> (x = y?=w602:bool)
    n266 = local read "fp"() -> (w619:fxp<+/-,20,10>)
    n267 = Greater?(x=w614, y="Dp_d_tol") -> (0:w613:bool)
    n268 = Select(t=w595, s=w602, f=w601) -> (s? t:f=w600:fxp<+/-,26,16>)
    n269 = Absolute Value(x=w619) -> (abs(x)=w620:fxp<+,20,10>)
    n270 = Select(t="fcp", s=w613, f="fstp") -> (s? t:f=w611:fxp<+/-,15,6>)
    n271 = Multiply(x=w620, y="fv_coeff. p") -> (x*y=w618:fxp<+/-,20,10>)
    n272 = Absolute Value(x=w601) -> (abs(x)=w608:fxp<+,25,15>)
    n273 = Sign(1:w600) -> (0:w599:fxp<+/-,2,2>)
    n274 = Multiply(x=w599, y="viscous_cons_p") -> (x*y=w604:fxp<+/-,20,10>)
    n275 = Multiply(x=w601, y="fvp") -> (x*y=w606:fxp<+/-,20,10>)
    n276 = Add(x=w611, y=w618) -> (x+y=w617:fxp<+/-,20,10>)
    n277 = Greater?(x=w608, y=fxp<+/-,25,15> 25.0) -> (0:w607:bool)
    n278 = Multiply(x=w599, y=w617) -> (x*y=w616:fxp<+/-,20,10>)
    n279 = Select(t=w604, s=w607, f=w606) -> (s? t:f=w605:fxp<+/-,20,10>)
    n280 = Add(x=w605, y=w616) -> (x+y=→"Friction comp_p":fxp<+/-,20,10>)
  }
  n281 = while "Friction compensation_y" {
    stop <- FALSE stop-if-true
    n282 = local read "Dy_d"() -> (w628:fxp<+/-,25,15>)
    n283 = local read "xy_d"() -> (w625:fxp<+/-,25,15>)
    n284 = Negate(x=w625) -> (-x=w624:fxp<+/-,26,16>)
    n285 = Absolute Value(x=w628) -> (abs(x)=w642:fxp<+,25,15>)
    n286 = Equal?(x=w628, y=fxp<+/-,25,15> 0.0) -> (x = y?=w629:bool)
    n287 = local read "fy"() -> (w648:fxp<+/-,20,10>)
    n288 = Select(t=w624, s=w629, f=w628) -> (s? t:f=w627:fxp<+/-,26,16>)
    n289 = Greater?(x=w642, y="Dy_d_tol") -> (0:w641:bool)
    n290 = Absolute Value(x=w648) -> (abs(x)=w649:fxp<+,20,10>)
    n291 = Multiply(x=w649, y="fv_coeff. y") -> (x*y=w646:fxp<+/-,20,10>)
    n292 = Select(t="fcy", s=w641, f="fsty") -> (s? t:f=w639:fxp<+/-,15,6>)
    n293 = Absolute Value(x=w628) -> (abs(x)=w636:fxp<+,25,15>)
    n294 = Sign(1:w627) -> (0:w626:fxp<+/-,2,2>)
    n295 = Multiply(x=w626, y="viscous_cons_y") -> (x*y=w631:fxp<+/-,20,10>)
    n296 = Multiply(x=w628, y="fvy") -> (x*y=w634:fxp<+/-,20,10>)
    n297 = Add(x=w639, y=w646) -> (x+y=w645:fxp<+/-,20,10>)
    n298 = Greater?(x=w636, y=fxp<+/-,25,15> 25.0) -> (0:w635:bool)
    n299 = Multiply(x=w626, y=w645) -> (x*y=w644:fxp<+/-,20,10>)
    n300 = Select(t=w631, s=w635, f=w634) -> (s? t:f=w633:fxp<+/-,20,10>)
    n301 = Add(x=w633, y=w644) -> (x+y=→"Friction comp_y":fxp<+/-,20,10>)
  }
  n302 = while "Gain comp_y" {
    shift-right: [w667] -> _
    shift-left: _ -> [w676]
    stop <- FALSE stop-if-true
    w663 = fxp<+,14,7> 111.8125  # 10^6/Mm^2/27
    w679 = fxp<+,14,7> 54.6015625  # 3*Mm
    n303 = local read "ky"() -> (w678:fxp<+,15,8>)
    n304 = Multiply(x=w676, y=fxp<+,12,-6> 0.00099945068359375) -> (x*y=w675:fxp<+,24,0>)
    n305 = Divide(x=w679, y=w678) -> (x/y=w674:fxp<+,23,7>)
    n306 = Multiply(x=w675, y=w674) -> (x*y=w673:fxp<+,32,0>)
    n307 = Square Root(x=w673) -> (sqrt(x)=w658:fxp<+,26,2>)
    n308 = local read "ky"() -> (w664:fxp<+,15,8>)
    n309 = Square(x=w658) -> (x^2=w666:fxp<+,27,3>)
    n310 = Select(t=w658, s="D_comp/tune_y", f="Kdy 2") -> (s? t:f=→"Kdy":fxp<+,34,10>)
    n311 = Square(x=w664) -> (x^2=w662:fxp<+,30,16>)
    n312 = local read "fy"() -> (w670:fxp<+/-,20,10>)
    n313 = Multiply(x=w666, y=w658) -> (x*y=w665:fxp<+,27,3>)
    n314 = Multiply(x=w662, y=w663) -> (x*y=w661:fxp<+,44,20>)
    n315 = Absolute Value(x=w670) -> (abs(x)=w671:fxp<+,20,10>)
    n316 = Multiply(x=w665, y=w661) -> (x*y=w656:fxp<+,27,10>)
    n317 = Multiply(x=w671, y="Kpy slope gain") -> (x*y=w669:fxp<+,12,4>)
    n318 = Add(x=w669, y="Kpy gain") -> (x+y=w667:fxp<+,12,6>)
    "Kpy" <- w667
    n319 = Select(t=w656, s="I_comp/tune_y", f="Kiy 2") -> (s? t:f=→"Kiy":fxp<+,27,10>)
  }
  n320 = while "ini" {
    stop <- FALSE stop-if-true
    n321 = case shown="True" "coe_ini" {
      frame False {
      }
      frame True {
        n322 = local write "fcp"(fxp<+/-,15,6> 6.0 ("fcp")) -> ()
        n323 = local write "Dp_d_tol"(fxp<+,20,12> 3.0 ("Dp_d_tol")) -> ()
        n324 = local write "tolerance_fy"(fxp<+,12,2> 1.0 ("tolerance_y")) -> ()
        n325 = local write "fstp"(fxp<+/-,15,6> 8.0 ("fstp")) -> ()
        n326 = local write "Kpp gain"(fxp<+,27,10> 3.0 ("Kpp gain")) -> ()
        n327 = local write "fcy"(fxp<+/-,15,6> 6.0 ("fcy")) -> ()
        n328 = local write "tolerance_fp"(fxp<+,12,2> 1.0 ("tolerance_p")) -> ()
        n329 = local write "AI loop wait (uSec)"(u8 20 ("AI loop wait (uSec)")) -> ()
        n330 = local write "AI diff loop wait (uSec) 2"(u32 500 ("AI diff loop wait (uSec) 2")) -> ()
        n331 = local write "fsty"(fxp<+/-,15,6> 12.0 ("fsty")) -> ()
        n332 = local write "Kpy gain"(fxp<+,27,10> 2.296875 ("Kpy gain")) -> ()
        n333 = local write "Dp stroke"(fxp<+,22,7> 30.0) -> ()
        n334 = local write "vq"(fxp<+/-,20,5> 0.0) -> ()
        n335 = local write "vd"(fxp<+/-,20,5> 5.0) -> ()
        n336 = local write "kp t"(fxp<+,15,8> 31.8046875 ("kp t")) -> ()
        n337 = local write "ky c"(fxp<+,15,8> 34.0234375 ("kp c")) -> ()
        n338 = local write "Dy_d_tol"(fxp<+,20,12> 0.1015625 ("Dy_d_tol")) -> ()
        n339 = local write "kp c"(fxp<+,15,8> 36.2421875 ("kp c")) -> ()
        n340 = local write "fvp"(fxp<+,20,12> 0.19921875 ("fvp")) -> ()
        n341 = local write "ky t"(fxp<+,15,8> 33.3359375 ("ky")) -> ()
        n342 = local write "fvy"(fxp<+,20,12> 0.19921875 ("fvy")) -> ()
        n343 = local write "fv_coeff. p"(fxp<+,13,1> 0.14990234375 ("fv_coeff. p")) -> ()
        n344 = local write "fv_coeff. y"(fxp<+,13,1> 0.14990234375 ("fv_coeff. y")) -> ()
        n345 = local write "Kpp slope gain"(fxp<+,20,1> 0.14999961853027344 ("Kpp slope gain")) -> ()
        n346 = local write "Kpy slope gain"(fxp<+,20,1> 0.14999961853027344 ("Kpy slope gain")) -> ()
      }
    }
  }
  n347 = while "Stiffness change_yp" {
    stop <- FALSE stop-if-true
    n348 = local read "x_p"() -> (w708:fxp<+/-,30,6>)
    n349 = local read "x_y"() -> (w718:fxp<+/-,30,6>)
    n350 = Less Than 0?(x=w708) -> (x < 0?=w709:bool)
    n351 = Less Than 0?(x=w718) -> (x < 0?=w717:bool)
    n352 = Select(t="kp c", s=w709, f="kp t") -> (s? t:f=w710:fxp<+,15,8>)
    n353 = Select(t="ky c", s=w717, f="ky t") -> (s? t:f=w716:fxp<+,15,8>)
    n354 = local write "kp"(w710) -> ()
    n355 = local write "ky"(w716) -> ()
  }
  n356 = while {
    shift-right: [w730] -> _
    shift-left: _ -> [w731]
    shift-right: [w723] -> _
    shift-left: fxp<+,36,6> 0.0 -> [w729]
    shift-right: [w721] -> _
    shift-left: _ -> [w722]
    stop <- FALSE stop-if-true
    n357 = call "Tick Count5"() -> ("Tick Count(uSec)"=w730:u8)
    n358 = Subtract(x=w730, y=w731) -> (x-y=w727:u8)
    n359 = To Fixed-Point(number=w727) -> (fixed-point=w726:fxp<+,8,8>)  [unwired: 1 in]
    n360 = Divide(x=w726, y=fxp<+,14,20> 1000000.0) -> (x/y=w725:fxp<+,15,-15>)
    n361 = Add(x=w725, y=w729) -> (x+y=w723:fxp<+,40,10>)
    n362 = Select(t=w723, s="Time_reset", f=w722) -> (s? t:f=w721:fxp<+,40,10>)
    n363 = Subtract(x=w723, y=w721) -> (x-y=→"time now":fxp<+/-,41,11>)
  }
